vi "Connect SV.vi"(0 "Axis Config in":T1, 11 "Error In":errorcluster) -> (4 "Axis Config out":T1, 6 "shared variable value change notification":refnum<user-event>, 8 "Shared Variables":refnum<k21>[](array[refnum]), 10 "Event Registration Refnum":refnum<event-registration>, 15 "Error Out":errorcluster)   [LabVIEW 2016, in "SMD-7615.lvlib"]
doc: "This VI connects Shared Variables to a User Event. The Event is triggerd at any Value change of the specified Shared Variables."
uses:
  SMD-7615.lvlib
  CTL/Stepper Drive Config.ctl
  CTL/SV General.ctl
  CTL/SV Inputs.ctl
  CTL/SV Outputs.ctl
  <vilib>/lvdsc/NI_DSC.lvlib
  <resource>/objmgr/ni.var.rc
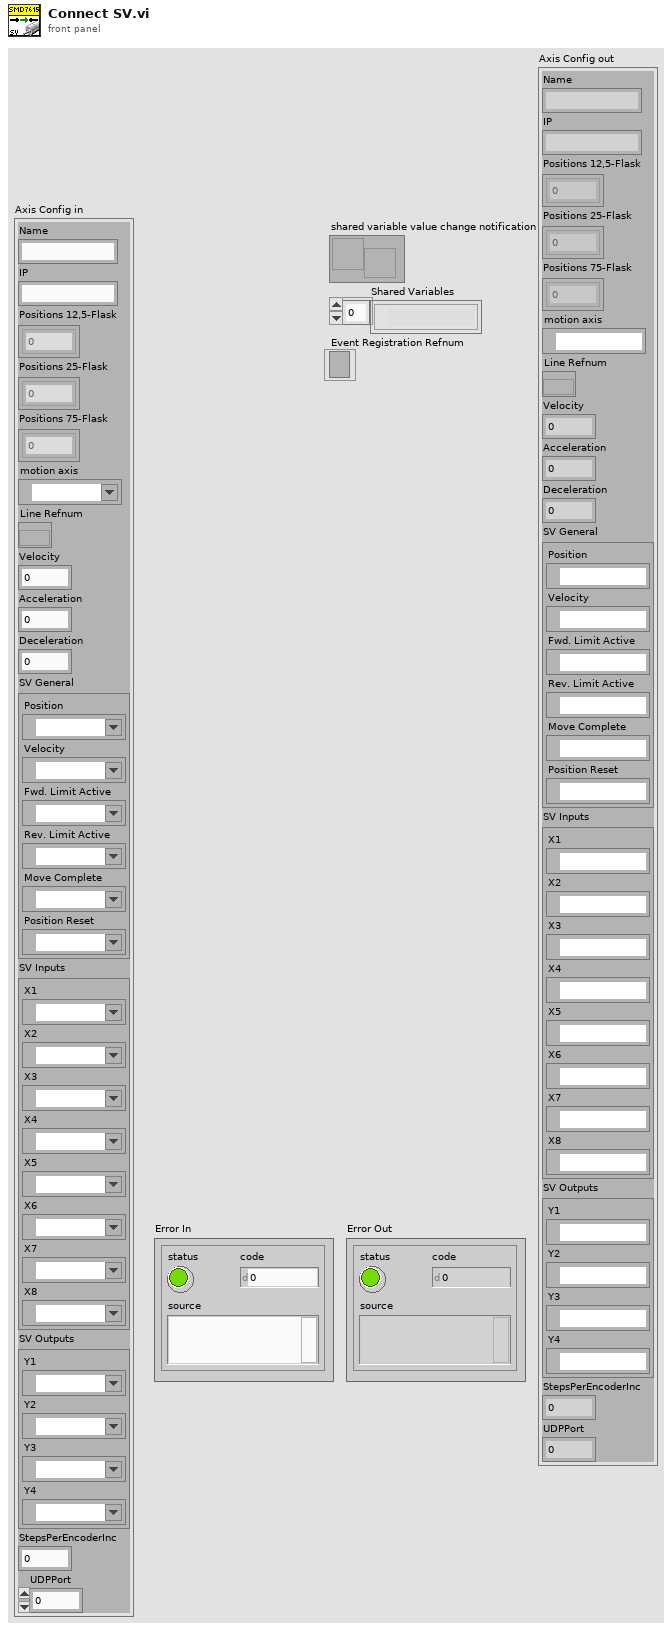
[diagram p1: front panel]
types:
  T1 = typedef "SMD-7615.lvlib/Stepper Drive Config.ctl" = cluster{"Name":string, "IP":string, "Positions 12,5-Flask":dbl[], "Positions 25-Flask":dbl[], "Positions 75-Flask":dbl[], "motion axis ":refnum<k21>, "Line Refnum":refnum<k20>, "Velocity":dbl, "Acceleration":dbl, "Deceleration":dbl, "SV General":T2, "SV Inputs":T3, "SV Outputs":T4, "StepsPerEncoderInc":i32, "UDPPort":u16}
  T2 = typedef "SMD-7615.lvlib/SV General.ctl" = cluster{"Position":refnum<k21>, "Velocity":refnum<k21>, "Fwd. Limit Active":refnum<k21>, "Rev. Limit Active":refnum<k21>, "Move Complete":refnum<k21>, "Position Reset":refnum<k21>}
  T3 = typedef "SMD-7615.lvlib/SV Inputs.ctl" = cluster{"X1":refnum<k21>, "X2":refnum<k21>, "X3":refnum<k21>, "X4":refnum<k21>, "X5":refnum<k21>, "X6":refnum<k21>, "X7":refnum<k21>, "X8":refnum<k21>}
  T4 = typedef "SMD-7615.lvlib/SV Outputs.ctl" = cluster{"Y1":refnum<k21>, "Y2":refnum<k21>, "Y3":refnum<k21>, "Y4":refnum<k21>}
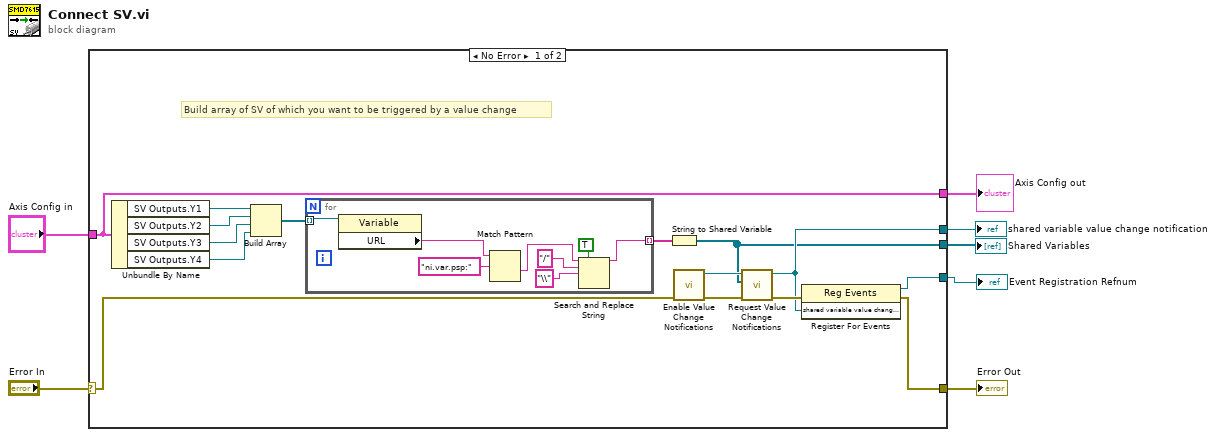
[diagram p0: block diagram]
diagram:
  n1 = case shown="No Error" "Error In" {
    selector: "Error In" -> [w13 w32]
    tunnel: "Axis Config in" -> [w11 w31]
    tunnel: [w12 w32] -> w5
    tunnel: [w11 w31] -> w4
    tunnel: [w10 _] -> w3
    tunnel: [w9 _] -> w2
    tunnel: [w8 _] -> w1
    frame No Error {
      # "Build array of SV of which you want to be triggered by a value change"
      n2 = Unbundle By Name(w11) -> ("SV Outputs.Y1"=w17:refnum<k21>, "SV Outputs.Y2"=w18:refnum<k21>, "SV Outputs.Y3"=w19:refnum<k21>, "SV Outputs.Y4"=w20:refnum<k21>)
      n3 = Build Array(w17, w18, w19, w20) -> (w21:refnum<k21>[])
      n4 = for {
        tunnel: w21 -> [w30] mode=indexing
        tunnel: [w23] -> w22 mode=indexing
        n5 = property class="Variable"(reference=w30) -> ("URL"=w28:string)  [unwired: 1 in, 2 out]
        n6 = Match Pattern(string=w28, regular expression="ni.var.psp:") -> (after substring=w24:string)  [unwired: 1 in, 3 out]
        n7 = Search and Replace String(replace all?=TRUE ("replace all? (F)"), input string=w24, search string="/", replace string="\\" ("replace string (\"\")")) -> (result string=w23:string)  [unwired: 4 in, 3 out]
      }
      n8 = String to Shared Variable(0:w22) -> (2:w9:refnum<k21>[])  [unwired: 1 out]
      n9 = call <vilib>:"Enable Value Change Notifications.vi"("error in (no error)"=w13) -> ("error out"=w14:errorcluster, "shared variable value change notification"=w15:refnum<user-event>)  [unwired: 9 out]
      n10 = call <vilib>:"Request Value Change Notifications.vi"("error in (no error)"=w14, "shared variables"=w9, "notification refnum"=w15) -> ("error out"=w16:errorcluster, "shared variable value change notification"=w10:refnum<user-event>)  [unwired: 1 in, 6 out]
      n11 = register-events(error in=w16, w10) -> (reference out=w8:refnum<event-registration>, error out=w12:errorcluster)  [unwired: 1 in]
    }
    frame Error {
    }
  }
  "Error Out" <- w5
  "Axis Config out" <- w4
  "shared variable value change notification" <- w3
  "Shared Variables" <- w2
  "Event Registration Refnum" <- w1
